vi "RichToFlatrfcontrol_GetDeviceTempsResponse.vi"(5 "OutputClusterType":T1, 11 "InputCluster":T3) -> (3 "OutputCluster":T1)   [LabVIEW 2024, in "FlexSDR_gRPC_client.lvlib"]
uses:
  rfcontrol_GetDeviceTempsResponse.ctl
  rfcontrol_TemperatureReadings.ctl
  rfcontrol_GetDeviceTempsResponse_Flat.ctl
  rfcontrol_TemperatureReadings_Flat.ctl
  FlexSDR_gRPC_client.lvlib
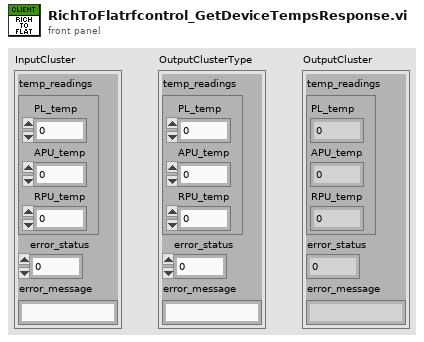
[diagram p1: front panel]
types:
  T1 = typedef "FlexSDR_gRPC_client.lvlib/rfcontrol_GetDeviceTempsResponse_Flat.ctl" = cluster{"temp_readings":T2, "error_status":i32, "error_message":string}
  T2 = typedef "FlexSDR_gRPC_client.lvlib/rfcontrol_TemperatureReadings_Flat.ctl" = cluster{"PL_temp":dbl, "APU_temp":dbl, "RPU_temp":dbl}
  T3 = typedef "FlexSDR_gRPC_client.lvlib/rfcontrol_GetDeviceTempsResponse.ctl" = cluster{"temp_readings":T4, "error_status":i32, "error_message":string}
  T4 = typedef "FlexSDR_gRPC_client.lvlib/rfcontrol_TemperatureReadings.ctl" = cluster{"PL_temp":dbl, "APU_temp":dbl, "RPU_temp":dbl}
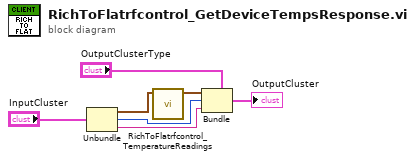
[diagram p0: block diagram]
diagram:
  n1 = Unbundle "Unbundle"("InputCluster") -> ("temp_readings"=w4:T4, "error_status"=w2:i32, "error_message"=w1:string)
  n2 = call "RichToFlatrfcontrol_TemperatureReadings.vi"("InputCluster"=w4) -> ("OutputCluster"=w3:T2)  [unwired: 10 in]
  n3 = Bundle "Bundle"(cluster="OutputClusterType", "temp_readings"=w3, "error_status"=w2, "error_message"=w1) -> (→"OutputCluster":T1)
